vi "RLC 电路频率特征曲线测量.vi"() -> ()   [LabVIEW 2021]
panel:
  out "Waveform Graph":dynamicdata(graph)
  out "相-频曲线 2":cluster{"Y":dbl[], "Y":dbl[]}[](graph)
  out "幅-频曲线 2":cluster{"Y":dbl[], "Y":dbl[]}[](graph)
  out "ω0":dbl
  in  "C/μF":dbl
  in  "L/mH":dbl
  in  "R/Ω":dbl
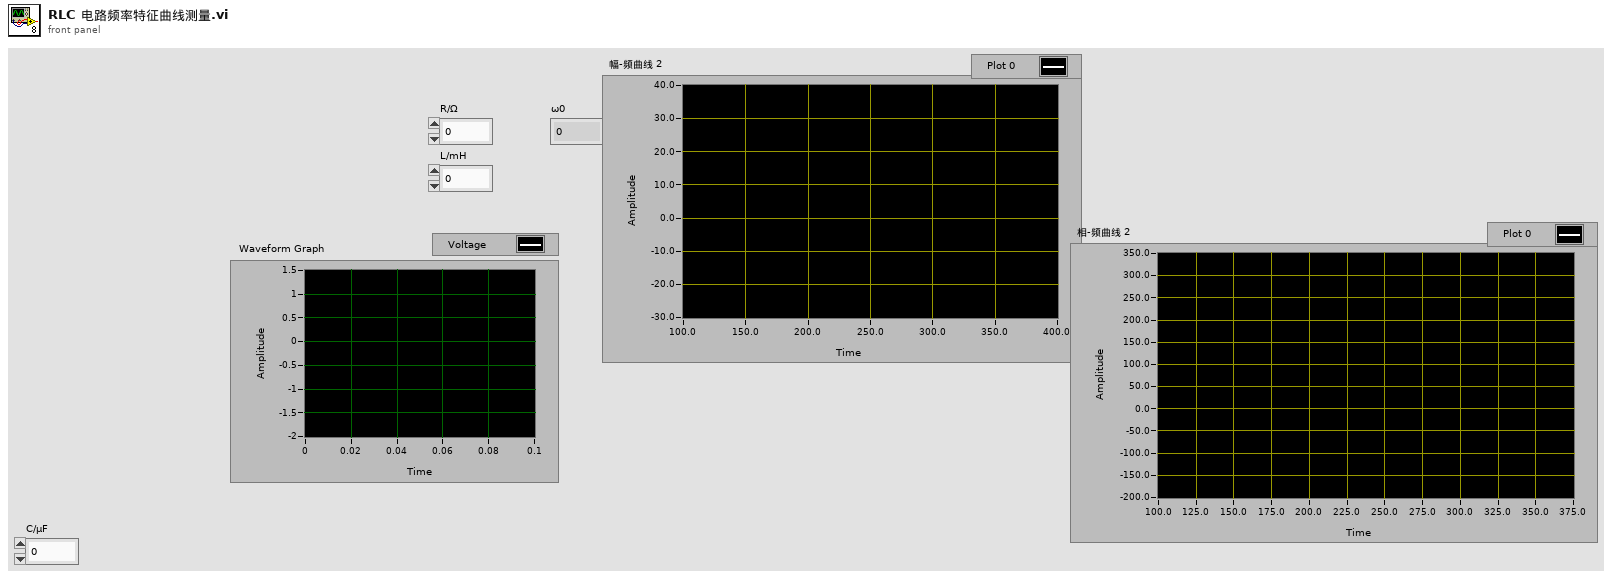
[diagram p1: front panel]
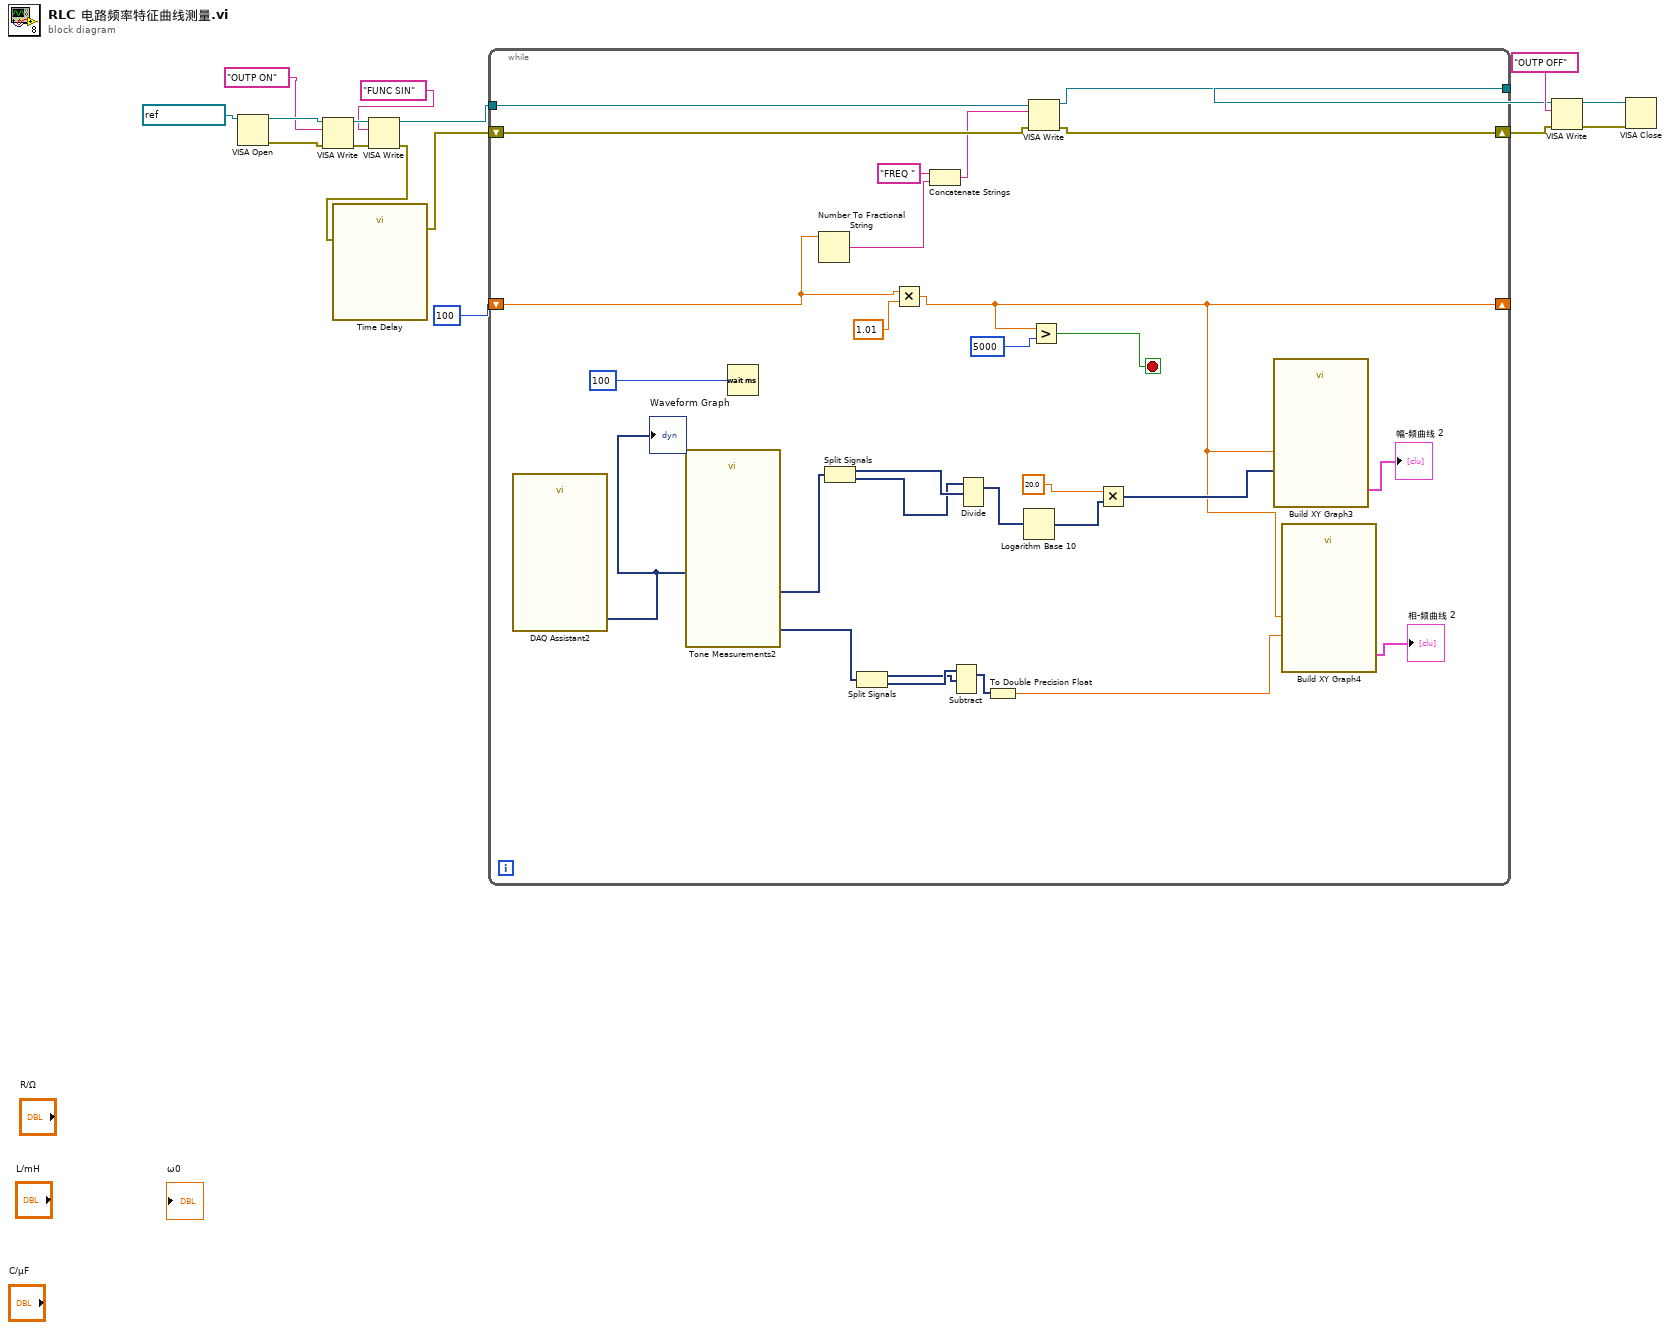
[diagram p0: block diagram]
diagram:
  n1 = VISA Open(VISA resource name=refnum<visa-resource-name> "DG1022U") -> (VISA resource name=w15:refnum<visa-resource-name>, error out=w14:errorcluster)  [unwired: 4 in]
  n2 = VISA Write(VISA resource name=w15, write buffer="OUTP ON", error in (no error)=w14) -> (VISA resource name out=w12:refnum<visa-resource-name>, error out=w10:errorcluster)  [unwired: 1 out]
  n3 = VISA Write(VISA resource name=w12, write buffer="FUNC SIN", error in (no error)=w10) -> (VISA resource name out=w6:refnum<visa-resource-name>, error out=w2:errorcluster)  [unwired: 1 out]
  n4 = call "Time Delay"("error in (no error)"=w2) -> ("error out"=w1:errorcluster)  [unwired: 10 in]
  n5 = while {
    tunnel: w6 -> [w44]
    tunnel: [w43] -> w5
    shift-right: [w41] -> w4
    shift-left: w1 -> [w42]
    shift-right: [w17] -> _
    shift-left: 100 -> [w35]
    stop <- w33 stop-if-true
    n6 = call "DAQ Assistant2"() -> ("data"=w22:dynamicdata)  [unwired: 17 in, 2 out]
    "Waveform Graph" <- w22
    n7 = call "Tone Measurements2"("Signals"=w22) -> ("Phase"=w21:dynamicdata, "Amplitude"=w20:dynamicdata)  [unwired: 7 in, 2 out]
    n8 = Wait (ms)(milliseconds to wait=u32 100) -> ()  [unwired: 1 out]
    n9 = Number To Fractional String(number=w35) -> (F-format string=w38:string)  [unwired: 3 in]
    n10 = Split Signals(w20) -> (w30:dynamicdata, w29:dynamicdata)  [unwired: 2 in]
    n11 = Split Signals(w21) -> (w27:dynamicdata, w28:dynamicdata)  [unwired: 2 in]
    n12 = Multiply(x=w35, y=1.01) -> (x*y=w17:dbl)
    n13 = Concatenate Strings("FREQ " ("string"), w38) -> (w40:string)
    n14 = Subtract(1:w27, 2:w28) -> (0:w19:dynamicdata)  [unwired: 1 in, 1 out]
    n15 = Divide(1:w30, 2:w29) -> (0:w24:dynamicdata)  [unwired: 1 in, 1 out]
    n16 = To Double Precision Float(number=w19) -> (double precision float=w18:dbl)
    n17 = Logarithm Base 10(1:w24) -> (0:w23:dynamicdata)
    n18 = VISA Write(VISA resource name=w44, write buffer=w40, error in (no error)=w42) -> (VISA resource name out=w43:refnum<visa-resource-name>, error out=w41:errorcluster)  [unwired: 1 out]
    n19 = Greater?(x=w17, y=5000) -> (0:w33:bool)
    n20 = Multiply(x=20.0, y=w23) -> (x*y=w25:dynamicdata)
    n21 = call "Build XY Graph3"("Y Input"=w25, "X Input"=w17) -> ("XY Graph"=→"幅-频曲线 2":cluster{"X":dbl[], "Y":dbl[]}[])  [unwired: 8 in, 1 out]
    n22 = call "Build XY Graph4"("Y Input"=w18, "X Input"=w17) -> ("XY Graph"=→"相-频曲线 2":cluster{"X":dbl[], "Y":dbl[]}[])  [unwired: 8 in, 1 out]
  }
  n23 = VISA Write(VISA resource name=w5, write buffer="OUTP OFF", error in (no error)=w4) -> (VISA resource name out=w8:refnum<visa-resource-name>, error out=w9:errorcluster)  [unwired: 1 out]
  n24 = VISA Close(VISA resource name=w8, error in (no error)=w9) -> ()  [unwired: 1 out]
